vi "Get Main Data.vi"(8 "error in (no error)":errorcluster caption="entrée d'erreur (pas d'erreur)", 11 "Database Altyor en entrée":refnum<class "Database Altyor Packaging.lvclass">) -> (0 "error out":errorcluster caption="sortie d'erreur", 2 "Main_Data Read":T1(array[cluster]), 3 "Database Altyor en sortie":refnum<class "Database Altyor Packaging.lvclass">)   [LabVIEW 2020, in "Library Instrument & Equipement.lvlib" / "Library Database.lvlib" / "Database Altyor Packaging.lvclass"]
uses:
  Database Altyor Packaging.lvclass
  Database Altyor Packaging.lvclass/Database Altyor Packaging.ctl
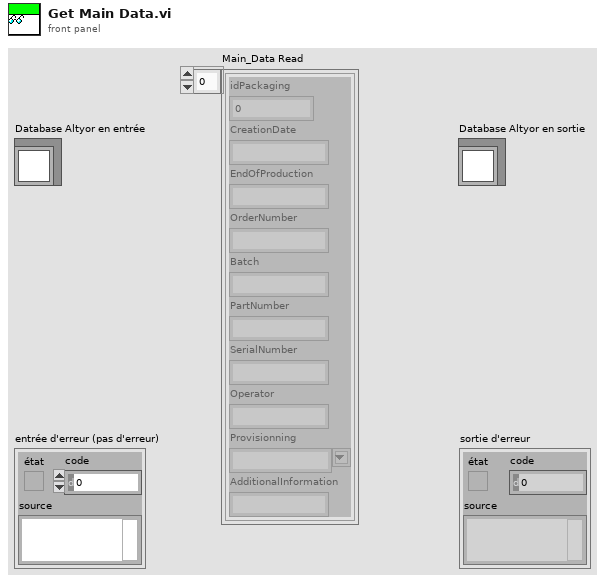
[diagram p1: front panel]
types:
  T1 = cluster{"idPackaging":u32, "CreationDate":string, "EndOfProduction":string, "OrderNumber":string, "Batch":string, "PartNumber":string, "SerialNumber":string, "Operator":string, "Provisionning":string, "AdditionalInformation":string}[]
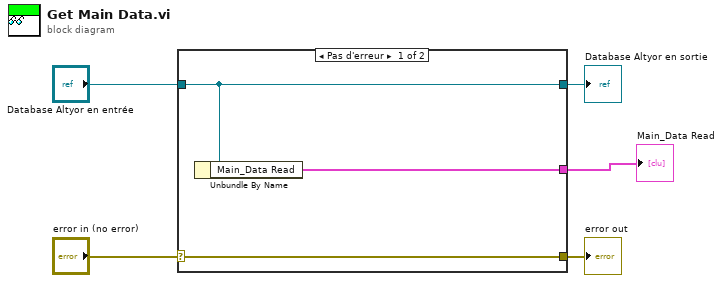
[diagram p0: block diagram]
diagram:
  n1 = case shown="Pas d'erreur" "error in (no error)" {
    selector: "error in (no error)" -> [w8 w9]
    tunnel: [w8 w9] -> w4
    tunnel: [w7 w10] -> w2
    tunnel: "Database Altyor en entrée" -> [w7 w10]
    tunnel: [w6 _] -> w1
    frame No Error {
      n2 = Unbundle By Name(w7) -> ("Main_Data Read"=w6:T1)
    }
    frame Error {
    }
  }
  "error out" <- w4
  "Database Altyor en sortie" <- w2
  "Main_Data Read" <- w1
